vi "main.vi"() -> ()   [LabVIEW 2019]
uses:
  <vilib>/Instr/_visa.llb/VISA Configure Serial Port (Instr).vi
panel:
  in  "Sham (trigger 4) upper":u32=15000
  in  "Ultrasound (trigger 3) upper":u32=8000
  in  "Questionnaire to sham":u32
  in  "Questionnaire to ultrasound":u32
  out "read buffer 2":string="trg ack\n"
  out "read buffer":string="set delay ack\n"
  in  "VISA resource name":refnum<visa-resource-name>="COM4"
  out "Abort trig":bool=TRUE
  out "Current trial index":u32=2
  out "Triggering...":bool=TRUE
  out "Download trigger\ndelay information":bool=TRUE
  out "Download US \nparameter to FG":bool=TRUE
  in  "stop trigger":bool
  in  "start trigger":bool
  in  "Number of ultrasonic\nor sham stimuli":u32=1
  in  "Inter-ultrasonic-stimulus\ninterval":u32=15
  in  "Sham (trigger 4)":u32=10000
  in  "Ultrasound (trigger 3)":u32=5000
  in  "Eye tracker (trigger 2)":u32
  in  "EEG (trigger 1)":u32
  # "ms"
  # "ms"
  # "ms"
  # "ms"
  # "ms"
  # "ms"
  # "sec"
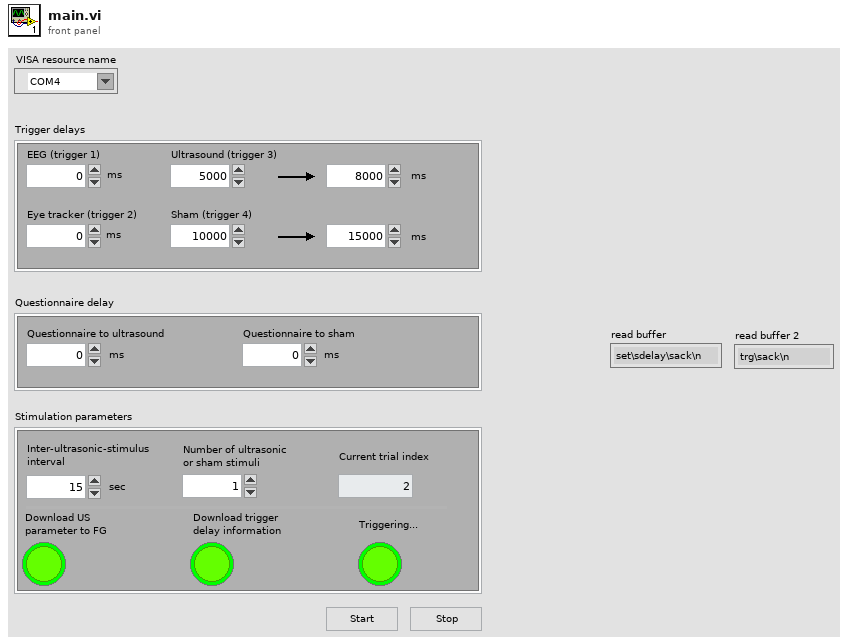
[diagram p1: front panel]
types:
  T1 = enum8{"Enabled", "Disabled", "Disabled and Grayed Out"}
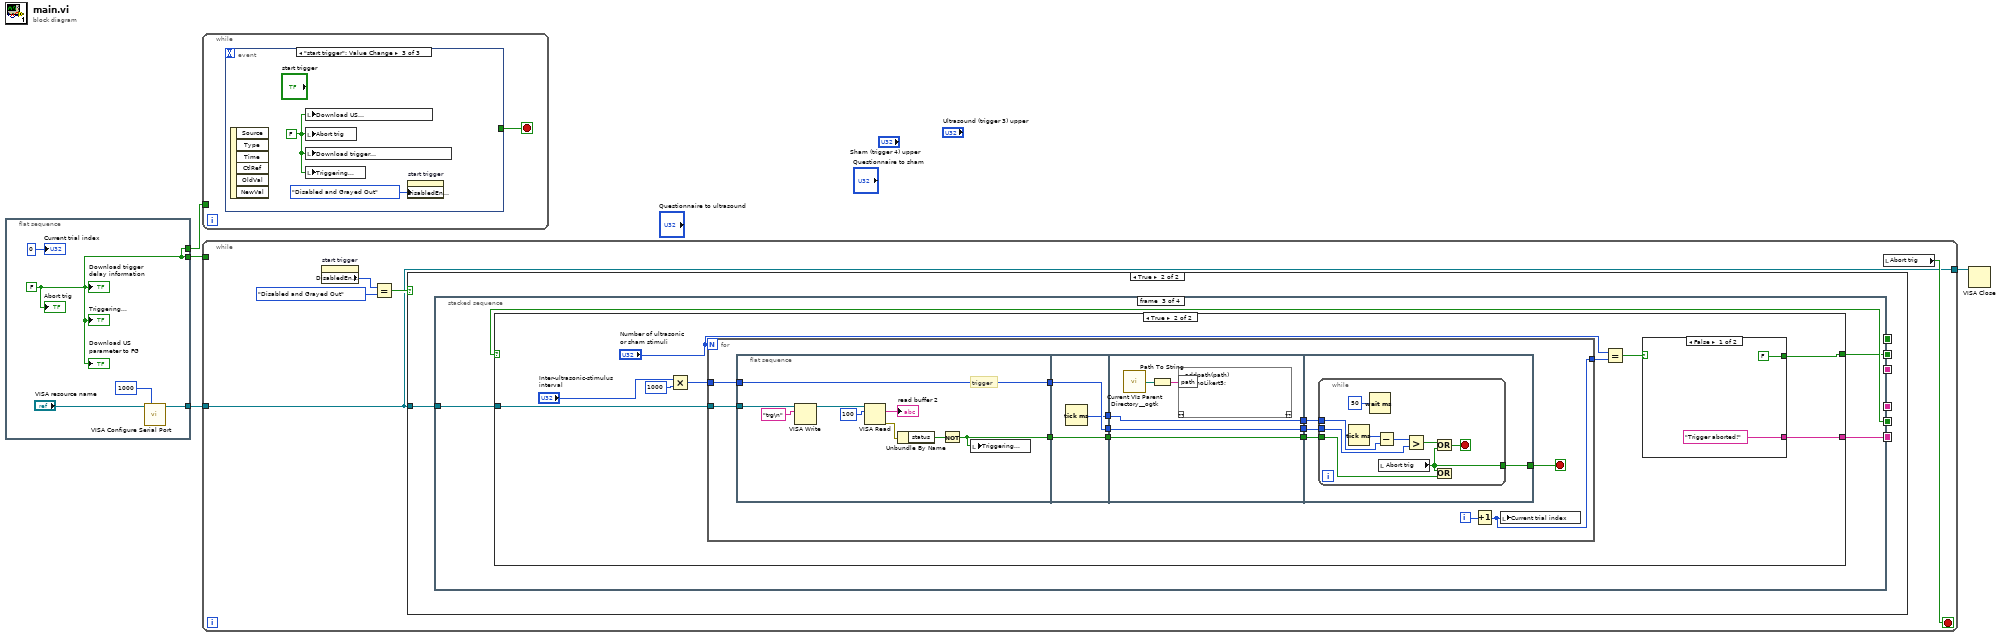
[diagram p0: block diagram]
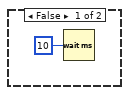
[diagram p2: hidden frame]
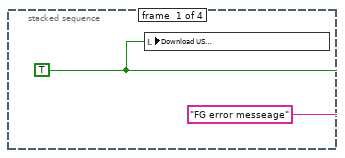
[diagram p3: hidden frame]
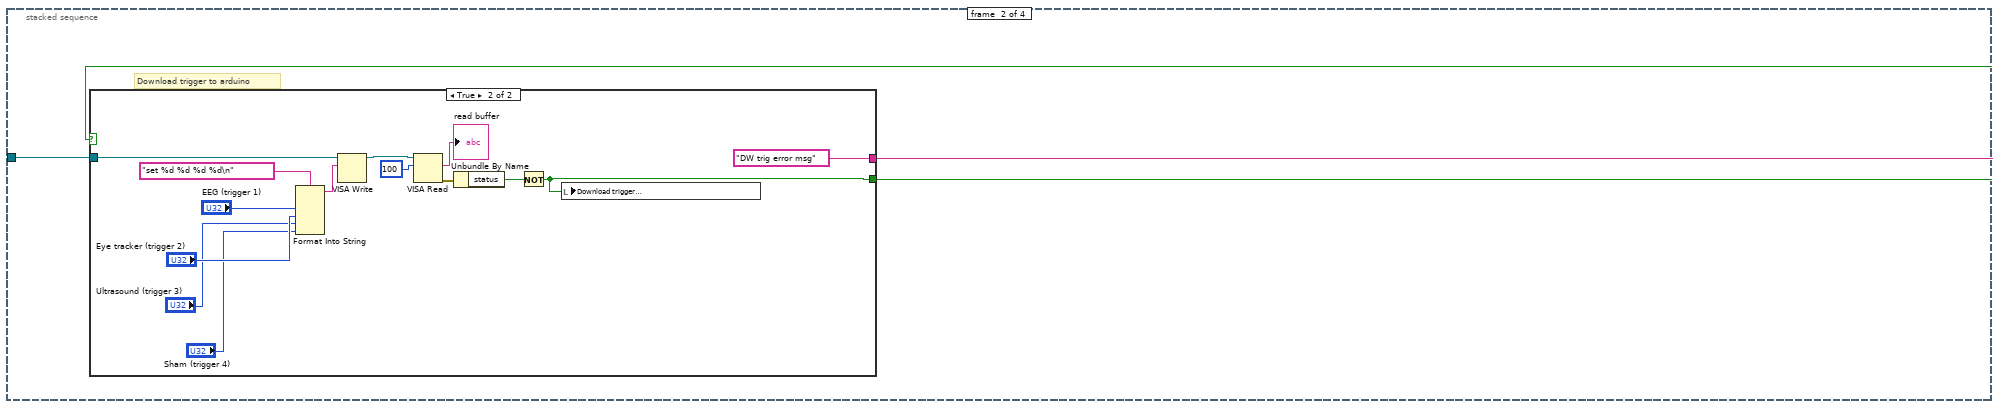
[diagram p4: hidden frame]
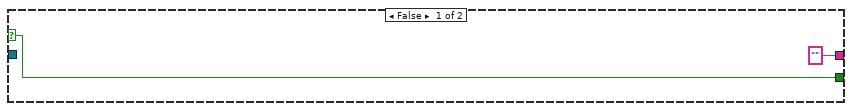
[diagram p5: hidden frame]
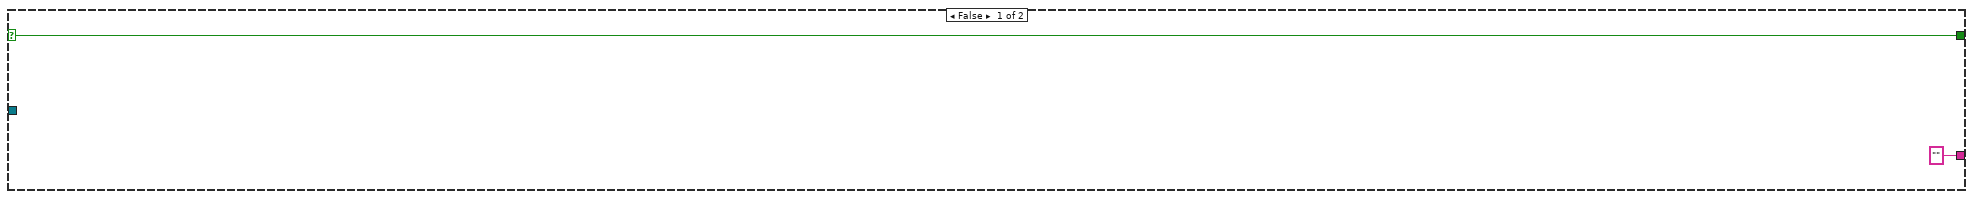
[diagram p6: hidden frame]
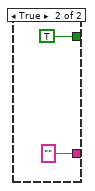
[diagram p7: hidden frame]
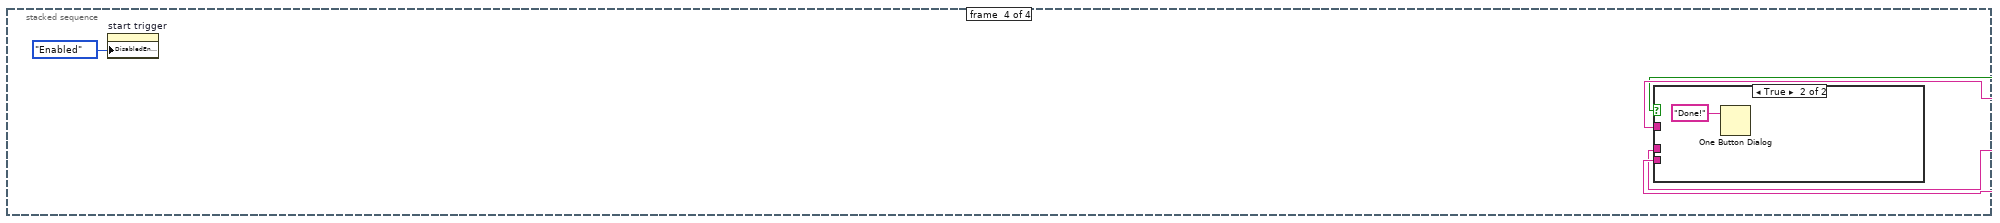
[diagram p8: hidden frame]
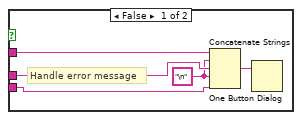
[diagram p9: hidden frame]
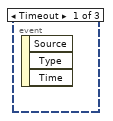
[diagram p10: hidden frame]
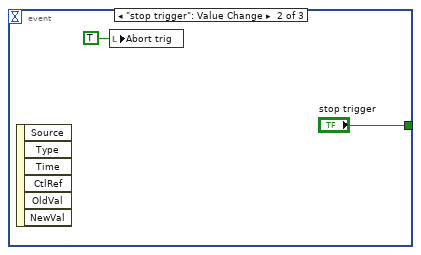
[diagram p11: hidden frame]
diagram:
  n1 = flat-sequence {
    tunnel: [w9] -> w4
    tunnel: [w9] -> w3
    tunnel: [w6] -> w2
    frame #0 {
      w9 = FALSE
      n2 = call-poly "VISA Configure Serial Port"("VISA resource name"="VISA resource name", "timeout (10sec)"=u32 1000) -> ("VISA resource name out"=w6:refnum<visa-resource-name>)  [unwired: 7 in, 6 out]
      "Download US \nparameter to FG" <- w9
      "Download trigger\ndelay information" <- w9
      "Triggering..." <- w9
      "Abort trig" <- w9
      "Current trial index" <- u32 0 ("Current trial index")
    }
  }
  n3 = while {
    tunnel: w4 -> [_]
    stop <- w10 stop-if-true
    n4 = event shown="[2] \"start trigger\": Value Change" {
      selector: _ -> [_ _ _]
      dyn-events: _ -> [_ _ _]
      timeout: _ -> [_ _ _]
      tunnel: [_ "stop trigger" _] -> w10
      event Timeout {
        n5 = event-data() -> ()  [unwired: 1 in, 3 out]
      }
      event "stop trigger": Value Change {
        n6 = event-data() -> ()  [unwired: 1 in, 6 out]
        n7 = local write "Abort trig"(TRUE ("Abort trig")) -> ()
      }
      event "start trigger": Value Change {
        w13 = FALSE
        n8 = event-data() -> ()  [unwired: 1 in, 6 out]
        n9 = local write "Download US \nparameter to FG"(w13) -> ()
        n10 = local write "Abort trig"(w13) -> ()
        n11 = local write "Download trigger\ndelay information"(w13) -> ()
        n12 = local write "Triggering..."(w13) -> ()
        n13 = property on="start trigger" class="Bool"("DisabledEnum"=T1."Disabled and Grayed Out" ("Disabled")) -> ()  [unwired: 2 in, 2 out]
      }
    }
  }
  n14 = while {
    tunnel: w3 -> [_]
    tunnel: w2 -> [w15]
    tunnel: [w15] -> w1
    stop <- w16 stop-if-true
    n15 = property on="start trigger" class="Bool"() -> ("DisabledEnum"=w19:T1)  [unwired: 2 in, 2 out]
    n16 = Equal?(x=w19, y=T1."Disabled and Grayed Out" ("Disabled")) -> (x = y?=w17:bool)
    n17 = case shown="True" w17 {
      tunnel: w15 -> [_ w21]
      frame False {
        n18 = Wait (ms)(milliseconds to wait=u32 10) -> ()  [unwired: 1 out]
      }
      frame True {
        n19 = stacked-sequence {
          seq-local: [w22 _ _ _] -> [_ w27 _ _]
          seq-local: [_ w26 _ _] -> [_ _ w47 _]
          seq-local: ["FG error messeage" _ _ _] -> [_ _ _ w110]
          seq-local: [_ w25 _ _] -> [_ _ _ w108]
          seq-local: [_ _ w46 _] -> [_ _ _ w109]
          seq-local: [_ _ w45 _] -> [_ _ _ w106]
          tunnel: w21 -> [_ w24 w44 _]
          frame #0 {
            w22 = TRUE
            n20 = local write "Download US \nparameter to FG"(w22) -> ()
          }
          frame #1 {
            # "Download trigger to arduino"
            n21 = case shown="True" w27 {
              selector: w27 -> [w29 _]
              tunnel: [w29 w30] -> w26
              tunnel: ["" "DW trig error msg"] -> w25
              tunnel: w24 -> [_ w37]
              frame False {
              }
              frame True {
                n22 = Format Into String(format string="set %d %d %d %d\n", "EEG (trigger 1)", "Eye tracker (trigger 2)", "Ultrasound (trigger 3)", "Sham (trigger 4)") -> (resulting string=w36:string)  [unwired: 2 in, 1 out]
                n23 = VISA Write(VISA resource name=w37, write buffer=w36) -> (VISA resource name out=w35:refnum<visa-resource-name>)  [unwired: 1 in, 2 out]
                n24 = VISA Read(VISA resource name=w35, byte count=u32 100) -> (read buffer=→"read buffer":string, error out=w32:errorcluster)  [unwired: 1 in, 2 out]
                n25 = Unbundle By Name(w32) -> ("status"=w31:bool)
                n26 = Not(x=w31) -> (.not. x?=w30:bool)
                n27 = local write "Download trigger\ndelay information"(w30) -> ()
              }
            }
          }
          frame #2 {
            n28 = case shown="True" w47 {
              selector: w47 -> [w48 _]
              tunnel: ["" w58] -> w46
              tunnel: [w48 w57] -> w45
              tunnel: w44 -> [_ w53]
              frame False {
              }
              frame True {
                n29 = Multiply(x="Inter-ultrasonic-stimulus\ninterval", y=u32 1000) -> (x*y=w54:u32)
                n30 = for {
                  N: "Number of ultrasonic\nor sham stimuli" -> [_]
                  tunnel: w54 -> [w72]
                  tunnel: w53 -> [w69]
                  tunnel: [w68] -> w52
                  i -> [w70]
                  stop <- w75 stop-if-true
                  n31 = flat-sequence {
                    tunnel: w72 -> [w84]
                    tunnel: [w84] -> w67
                    tunnel: [w76] -> w65
                    tunnel: w69 -> [w78]
                    tunnel: w67 -> [w87]
                    tunnel: [w87] -> w66
                    tunnel: w65 -> [w86]
                    tunnel: [w86] -> w64
                    tunnel: [w85] -> w63
                    tunnel: w66 -> [w92]
                    tunnel: [w92] -> w74
                    tunnel: [w88] -> w73
                    tunnel: [w91] -> w71
                    tunnel: w64 -> [w91]
                    tunnel: w63 -> [w88]
                    tunnel: [w95] -> w75
                    tunnel: w74 -> [w96]
                    tunnel: w73 -> [w94]
                    tunnel: w71 -> [w93]
                    frame #0 {
                      # "trigger"
                      n32 = VISA Write(VISA resource name=w78, write buffer="trg\n") -> (VISA resource name out=w83:refnum<visa-resource-name>)  [unwired: 1 in, 2 out]
                      n33 = VISA Read(VISA resource name=w83, byte count=u32 100) -> (read buffer=→"read buffer 2":string, error out=w80:errorcluster)  [unwired: 1 in, 2 out]
                      n34 = Unbundle By Name(w80) -> ("status"=w79:bool)
                      n35 = Not(x=w79) -> (.not. x?=w76:bool)
                      n36 = local write "Triggering..."(w76) -> ()
                    }
                    frame #1 {
                      n37 = Tick Count (ms)() -> (millisecond timer value=w85:u32)
                    }
                    frame #2 {
                      n38 = call <userlib>:"Current VIs Parent Directory__ogtk.vi"() -> ("Parent Directory (+ Relative)"=w90:path)  [unwired: 5 in]
                      n39 = Path To String(path=w90) -> (string=w89:string)
                      n40 = script code="addpath(path)\nDemoLikert5;"("path"=w89) -> ()  [unwired: 1 in, 1 out]
                    }
                    frame #3 {
                      n41 = while {
                        tunnel: w96 -> [w101]
                        tunnel: [w97] -> w95
                        tunnel: w94 -> [w103]
                        tunnel: w93 -> [w98]
                        stop <- w100 stop-if-true
                        n42 = Tick Count (ms)() -> (millisecond timer value=w104:u32)
                        n43 = Wait (ms)(milliseconds to wait=u32 50) -> ()  [unwired: 1 out]
                        n44 = Subtract(x=w104, y=w103) -> (x-y=w102:u32)
                        n45 = local read "Abort trig"() -> (w97:bool)
                        n46 = Greater?(x=w102, y=w101) -> (0:w99:bool)
                        n47 = Or(x=w99, y=w97) -> (x .or. y?=w100:bool)
                        n48 = Or(x=w97, y=w98) -> ()  [unwired: 1 out]
                      }
                    }
                  }
                  n49 = Increment(x=w70) -> (x+1=w68:i32)
                  n50 = local write "Current trial index"(w68) -> ()
                }
                n51 = Equal?(x="Number of ultrasonic\nor sham stimuli", y=w52) -> (x = y?=w50:bool)
                n52 = case shown="False" w50 {
                  tunnel: ["Trigger aborted!" ""] -> w58
                  tunnel: [FALSE TRUE] -> w57
                  frame False {
                  }
                  frame True {
                  }
                }
              }
            }
          }
          frame #3 {
            n53 = property on="start trigger" class="Bool"("DisabledEnum"=T1."Enabled" ("Disabled")) -> ()  [unwired: 2 in, 2 out]
            n54 = case shown="True" w106 {
              tunnel: w110 -> [w115 _]
              tunnel: w109 -> [w113 _]
              tunnel: w108 -> [w112 _]
              frame False {
                w111 = "\n" ("string")
                # "Handle error message"
                n55 = Concatenate Strings(w115, w111, w112, w111, w113) -> (w114:string)
                n56 = One Button Dialog(message=w114) -> ()  [unwired: 1 in, 1 out]
              }
              frame True {
                n57 = One Button Dialog(message="Done!") -> ()  [unwired: 1 in, 1 out]
              }
            }
          }
        }
      }
    }
    n58 = local read "Abort trig"() -> (w16:bool)
  }
  n59 = VISA Close(VISA resource name=w1) -> ()  [unwired: 1 in, 1 out]
